vi "1_2_Periodicity of discrete sinusoids.vi"() -> ()   [LabVIEW 2009]
panel:
  out "String":string
  in  "?":dbl=0.7999999999999997 min=0.0 step=0.01
  out "?":dbl[](graph)=[1.0, -0.8090169943749469, 0.30901699437494556, 0.3090169943749502, -0.8090169943749498, 1.0, -0.8090169943749439, 0.30901699437494, 0.30901699437495495, -0.8090169943749521, 1.0, -0.8090169943749406, 0.3090169943749362, 0.30901699437496216, -0.8090169943749566, 1.0, -0.8090169943749381, 0.30901699437493235, 0.3090169943749626, -0.8090169943749569, 1.0, -0.8090169943749337, 0.3090169943749251, 0.3090169943749698, -0.8090169943749613, 1.0, -0.8090169943749292, 0.30901699437491786, 0.30901699437497704, -0.8090169943749658, 1.0, -0.8090169943749289, 0.3090169943749174, 0.30901699437497754, -0.8090169943749661, 1.0, -0.8090169943749287, 0.3090169943749169, 0.309016994374978, -0.8090169943749663]
  in  "?":dbl=1.1999999999999997 min=0.0 step=0.01
  out "?":dbl[](graph)=[1.0, -0.809016994374948, 0.3090169943749494, 0.3090169943749436, -0.809016994374945, 1.0, -0.8090169943749521, 0.30901699437495517, 0.30901699437493957, -0.8090169943749425, 1.0, -0.8090169943749526, 0.3090169943749626, 0.3090169943749321, -0.8090169943749379, 1.0, -0.8090169943749571, 0.3090169943749701, 0.3090169943749314, -0.8090169943749332, 1.0, -0.8090169943749618, 0.309016994374964, 0.3090169943749239, -0.8090169943749287, 1.0, -0.8090169943749663, 0.3090169943749715, 0.3090169943749165, -0.8090169943749324, 1.0, -0.8090169943749627, 0.3090169943749789, 0.30901699437490904, -0.8090169943749195, 1.0, -0.8090169943749672, 0.30901699437498636, 0.30901699437490154, -0.8090169943749316]
  in  "stop":bool
  # "Program Developed by Indranil Sinharoy"
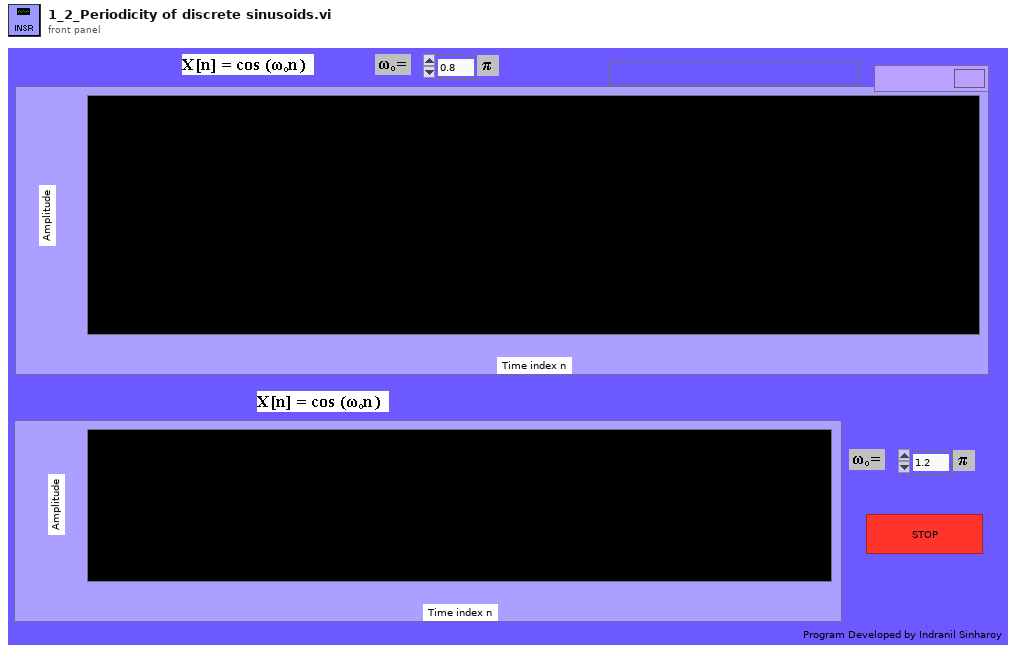
[diagram p1: front panel]
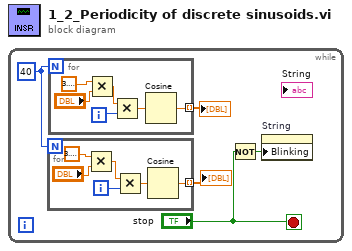
[diagram p0: block diagram]
diagram:
  n1 = while {
    stop <- "stop" stop-if-true
    w3 = 40
    n2 = for {
      N: w3 -> [_]
      tunnel: [w11] -> w4 mode=indexing
      i -> [w8]
      n3 = Multiply(x=3.141592653589793, y="?") -> (x*y=w9:dbl)
      n4 = Multiply(x=w9, y=w8) -> (x*y=w7:dbl)
      n5 = Cosine(x=w7) -> (cos(x)=w11:dbl)
    }
    "?" <- w4
    n6 = for {
      N: w3 -> [_]
      tunnel: [w17] -> w5 mode=indexing
      i -> [w14]
      n7 = Multiply(x=3.141592653589793, y="?") -> (x*y=w15:dbl)
      n8 = Multiply(x=w15, y=w14) -> (x*y=w13:dbl)
      n9 = Cosine(x=w13) -> (cos(x)=w17:dbl)
    }
    "?" <- w5
    n10 = Not(x="stop") -> (.not. x?=w2:bool)
    n11 = property on="String" class="Str"("Blinking"=w2) -> ()  [unwired: 2 in, 2 out]
  }
